vi "Write FIFO.vi"(8 "error in (no error)":errorcluster, 9 "timeout in ms (0)":i32 format="%d ms", 10 "element":i32, 11 "Pool in":refnum<class "Pool.lvclass">) -> (0 "error out":errorcluster, 1 "timed out?":bool, 3 "Pool out":refnum<class "Pool.lvclass">)   [LabVIEW 2017, in "DSF Core.lvlib" / "Pool.lvclass"]
uses:
  Pool.lvclass
  Pool.lvclass/Pool.ctl
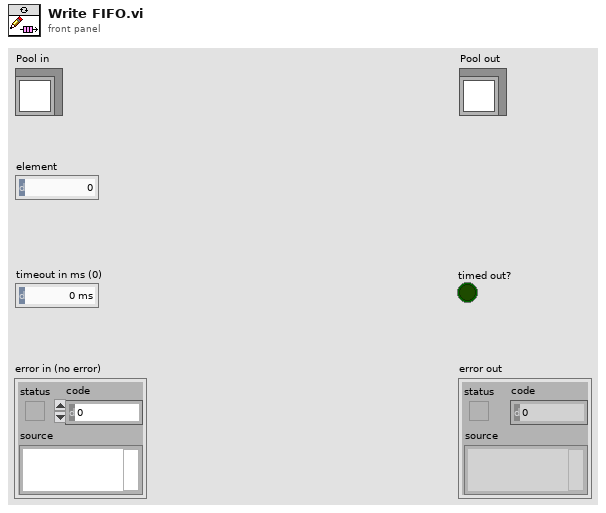
[diagram p1: front panel]
types:
  T1 = typedef "DSF Core.lvlib/FIFO Flags.ctl" = cluster{"Infinite Timeouts":bool}
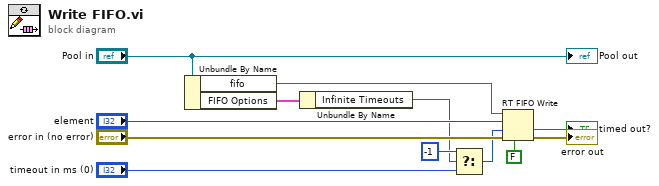
[diagram p0: block diagram]
diagram:
  n1 = Unbundle By Name("Pool in") -> ("fifo"=w2:refnum<k33>, "FIFO Options"=w4:T1)
  n2 = Unbundle By Name(w4) -> ("Infinite Timeouts"=w3:bool)
  n3 = Select(t=-1, s=w3, f="timeout in ms (0)") -> (s? t:f=w5:i32)
  n4 = RT FIFO Write(0:w2, 1:"element", 2:w5, 3:"error in (no error)", 5:FALSE ("overwrite on timeout (T)")) -> (10:→"timed out?":bool, 11:→"error out":errorcluster)  [unwired: 2 out]
  "Pool out" <- "Pool in"
